vi "Initialize Analysis.vi"(8 "error in (no error)":errorcluster, 11 "WaveformProcessor in":refnum<class "WaveformProcessor.lvclass">) -> (0 "error out":errorcluster, 3 "WaveformProcessor out":refnum<class "WaveformProcessor.lvclass">)   [LabVIEW 2019, in "Variant Parser.lvlib" / "WaveformProcessor.lvclass"]
uses:
  Library/WaveformProcessor.lvclass
  Custom Controls/Pulse Analysis.ctl
  Library/WaveformProcessor.lvclass/WaveformProcessor.ctl
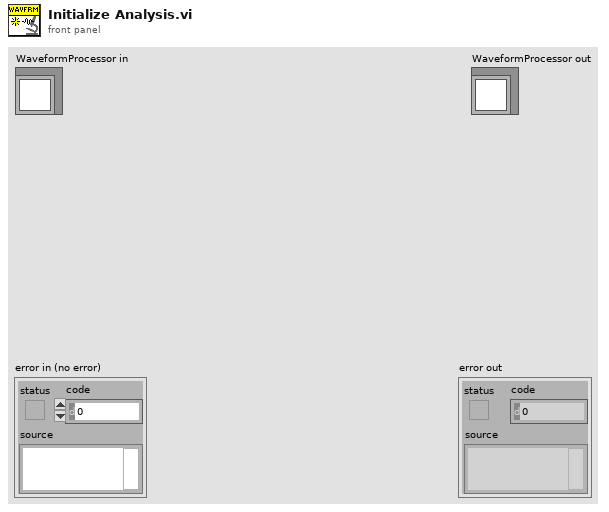
[diagram p1: front panel]
types:
  T1 = typedef "Variant Parser.lvlib/WaveformProcessor.lvclass/Pulse Analysis.ctl" = cluster{"tpulseStart":dbl, "tpulseEnd":dbl, "RisingSlope":dbl, "FallingSlope":dbl, "tHoldoff":dbl, "PeakAmplitude":dbl, "PulseAmplitude":dbl, "tpulse":dbl, "tPulseRise":dbl, "tPulseFall":dbl}
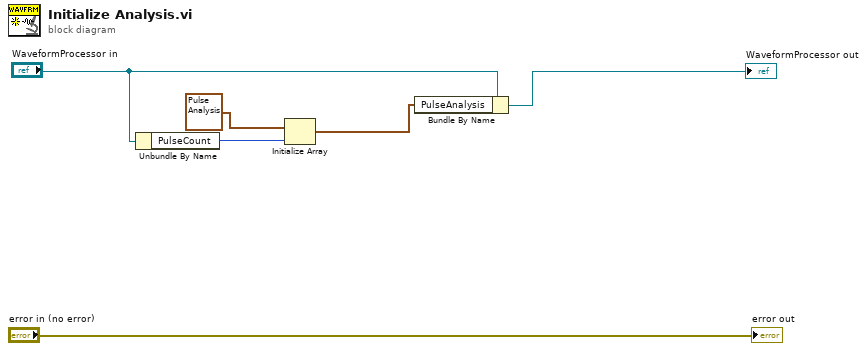
[diagram p0: block diagram]
diagram:
  n1 = Unbundle By Name("WaveformProcessor in") -> ("PulseCount"=w6:i32)
  n2 = Initialize Array(T1 {"tpulseStart"=0.0, "tpulseEnd"=0.0, "RisingSlope"=0.0, "FallingSlope"=0.0, "tHoldoff"=0.0, "PeakAmplitude"=0.0, "PulseAmplitude"=0.0, "tpulse"=0.0, "tPulseRise"=0.0, "tPulseFall"=0.0} ("PulseAnalysis"), w6) -> (w4:T1[])
  n3 = Bundle By Name(cluster="WaveformProcessor in", "PulseAnalysis"=w4) -> (→"WaveformProcessor out":refnum<class "WaveformProcessor.lvclass">)
  "error out" <- "error in (no error)"
